vi "New Queue Transport.vi"(10 "Max Queue Size (-1)":i32=-1) -> (0 "error out":errorcluster, 3 "QueueTransport":refnum<class "QueueTransport.lvclass">)   [LabVIEW 2017, in "Transport.lvlib" / "QueueTransport.lvclass"]
doc: "<License>\nCopyright © 2017 Composed Systems, LLC | All rights reserved\nwww.composed.io\n\nAuthor: Ethan Stern <ethan.stern@composed.io>\n\nThis software is provided \"AS IS\" WITHOUT WARRANTIES, either express or implied, AND IS FOR EDUCATIONAL PURPOSES ONLY.\n</License>"
uses:
  QueueTransport.lvclass
  QueueTransport.lvclass/QueueTransport.ctl
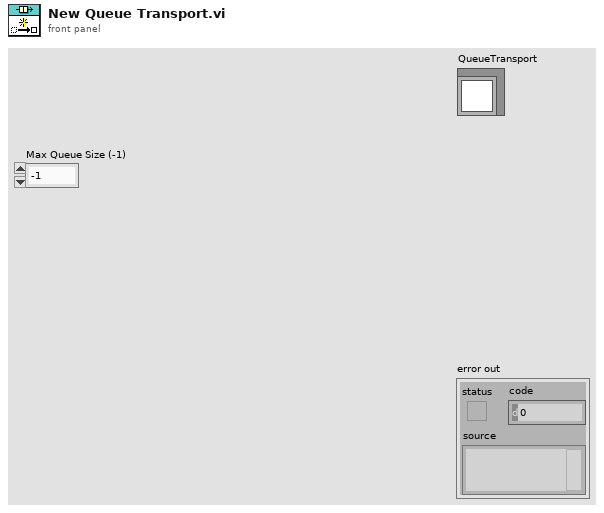
[diagram p1: front panel]
types:
  T1 = cluster{"Data":variant, "Publication Time":timestamp}
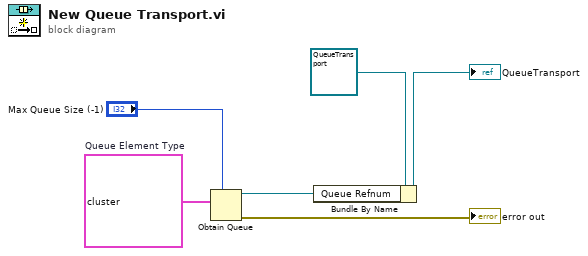
[diagram p0: block diagram]
diagram:
  w2 = T1 {"Data"=variant, "Publication Time"=timestamp(0 s since 1904-01-01)}  # Queue Element Type
  n1 = Obtain Queue(max queue size (-1, unlimited)="Max Queue Size (-1)", element data type=w2) -> (queue out=w1:refnum<queue>, error out=→"error out":errorcluster)  [unwired: 3 in, 1 out]
  n2 = Bundle By Name(cluster=refnum<class "QueueTransport.lvclass"> refnum ("ActorMessage in"), "Queue Refnum"=w1) -> (→"QueueTransport":refnum<class "QueueTransport.lvclass">)
